vi "Prepare Inputs.vi"(7 "SMO":refnum<class "SMO.lvclass">, 8 "error in (no error)":errorcluster, 10 "Inputs":variant[](array[variant]), 11 "API":T1) -> (0 "error out":errorcluster, 3 "API dup":T1)   [LabVIEW 2019, in "SMOFacade.lvclass"]
doc: "JKI State Machine Objects (SMO) 1.3.0.56\nJKI - JKI\nCopyright (c) 2017, JKI"
uses:
  SMOFacade.lvclass
  Registry/SMO_API--Cluster.ctl
  Terminal/Terminal.lvclass
  SMO/SMO.lvclass
  Registry/Registry-SMO.lvclass
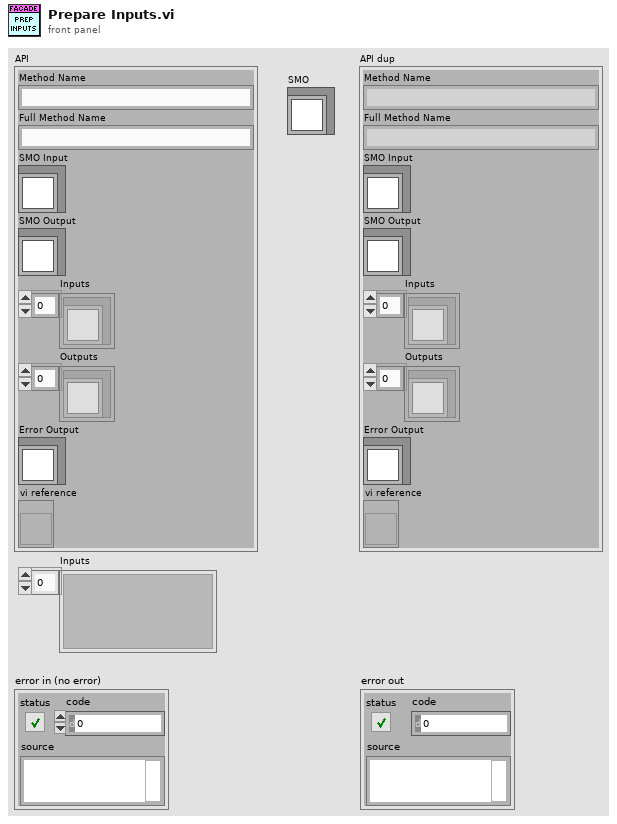
[diagram p1: front panel]
types:
  T1 = typedef "Registry-SMO.lvclass/SMO_API--Cluster.ctl" = cluster{"Method Name":string, "Full Method Name":string, "SMO Input":refnum<class "Terminal.lvclass">, "SMO Output":refnum<class "Terminal.lvclass">, "Inputs":refnum<class "Terminal.lvclass">[], "Outputs":refnum<class "Terminal.lvclass">[], "Error Output":refnum<class "Terminal.lvclass">, "vi reference":refnum<vi>}
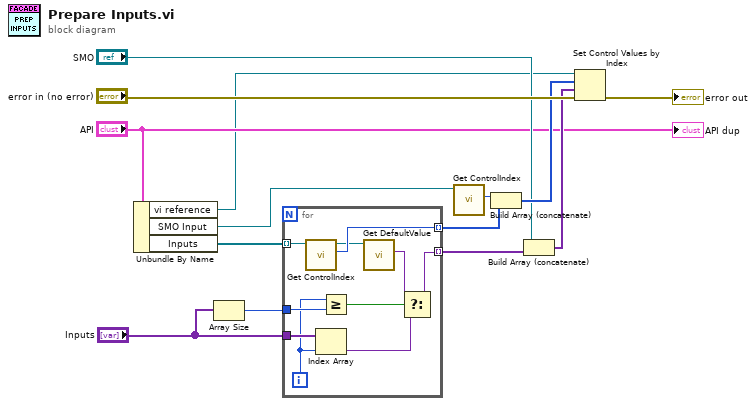
[diagram p0: block diagram]
diagram:
  n1 = Unbundle By Name("API") -> ("vi reference"=w3:refnum<vi>, "SMO Input"=w12:refnum<class "Terminal.lvclass">, "Inputs"=w6:refnum<class "Terminal.lvclass">[])
  n2 = Array Size(array="Inputs") -> (size(s)=w1:i32)
  n3 = for {
    tunnel: w6 -> [w24] mode=indexing
    tunnel: [w23] -> w11 mode=indexing
    tunnel: [w15] -> w10 mode=indexing
    tunnel: "Inputs" -> [w21]
    tunnel: w1 -> [w20]
    i -> [w19]
    n4 = call "Get ControlIndex.vi"("Terminal in"=w24) -> ("ControlIndex"=w23:i32, "Terminal out"=w22:refnum<class "Terminal.lvclass">)  [unwired: 8 in, 1 out]
    n5 = Index Array(array=w21, index=w19) -> (element=w17:variant)
    n6 = Greater Or Equal?(x=w19, y=w20) -> (x >= y?=w18:bool)
    n7 = call "Get DefaultValue.vi"("Terminal in"=w22) -> ("Default Value"=w16:variant)  [unwired: 7 in, 3 out]
    n8 = Select(t=w16, s=w18, f=w17) -> (s? t:f=w15:variant)
  }
  n9 = call "Get ControlIndex.vi"("Terminal in"=w12) -> ("ControlIndex"=w13:i32)  [unwired: 8 in, 2 out]
  n10 = Build Array (concatenate)(w13, w11) -> (w8:i32[])
  n11 = Build Array (concatenate)("SMO", w10) -> (w9:variant[])
  n12 = Set Control Values by Index(0:w3, 1:w8, 2:w9, 3:"error in (no error)") -> (11:→"error out":errorcluster)
  "API dup" <- "API"
